vi "Create Instrument.vi"(8 "error in (no error)":errorcluster, 10 "name":string, 11 "Instrument.SR7270 in":refnum<class "Instrument.SR7270.lvclass">) -> (0 "error out":errorcluster, 3 "Instrument.SR7270 out":refnum<class "Instrument.SR7270.lvclass">)   [LabVIEW 2016, in "Instrument.SR7270.lvclass"]
uses:
  Instrument.SR7270.lvclass
  levylab_inst/lvsrc/SMOs/Instrument/Instrument.lvclass
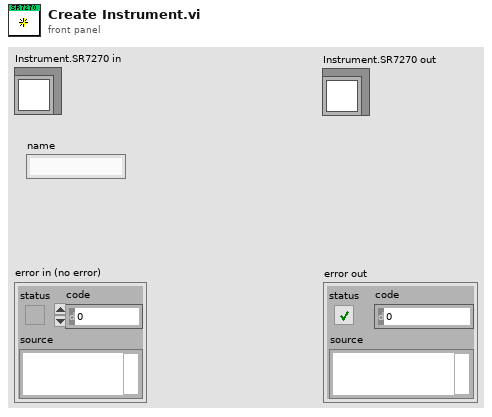
[diagram p1: front panel]
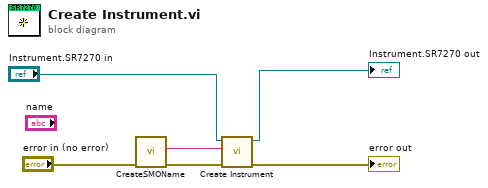
[diagram p0: block diagram]
diagram:
  n1 = call "CreateSMOName.vi"("error in (no error)"="error in (no error)") -> ("error out"=w1:errorcluster, "Name"=w2:string)  [unwired: 9 in]
  n2 = call-parent "Create Instrument.vi"("error in (no error)"=w1, "name"=w2, "Instrument in"="Instrument.SR7270 in") -> ("error out"=→"error out":errorcluster, "Instrument out"=→"Instrument.SR7270 out":refnum<class "Instrument.SR7270.lvclass">)  [unwired: 7 in]
